vi "PE Close.vi"(8 "error in (no error)":errorcluster, 11 "peHandle":u32) -> (0 "error out":errorcluster, 3 "function return":i32)   [LabVIEW 2011, in "libPhyspec.lvlib"]
doc: "PHYSPEC_API PE_STATUS PE_Close(PE_HANDLE peHandle);"
uses:
  libPhyspec.lvlib
  libPhyspec.dll
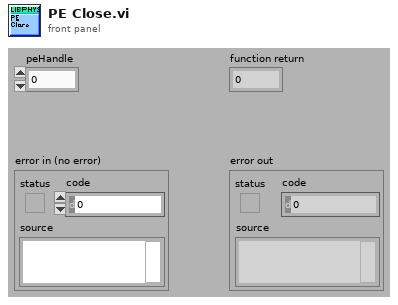
[diagram p1: front panel]
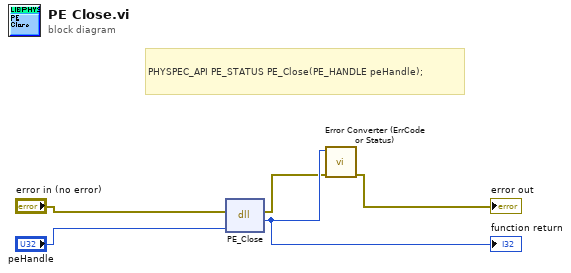
[diagram p0: block diagram]
diagram:
  # "PHYSPEC_API PE_STATUS PE_Close(PE_HANDLE peHandle);"
  n1 = dll-call lib="D:/users/nicolas/PHySpec-SDK-1.0.0/Labview-example/libPhyspec/libPhyspec.*" fn="PE_Close"(error in="error in (no error)", "peHandle"="peHandle") -> (error out=w2:errorcluster, "return type"=w5:i32)  [unwired: 3 in, 1 out]
  "function return" <- w5
  n2 = call "Error Converter (ErrCode or Status).vi"("error in (no error)"=w2, "error code"=w5) -> ("error out"=→"error out":errorcluster)  [unwired: 9 in]
